vi "Pnuematic_Initialization.vi"   [LabVIEW 2018]
uses:
  <vilib>/Rock Robotics/WPI/Solenoid/WPI_SolenoidChannel.ctl
  <vilib>/Rock Robotics/WPI/Solenoid/WPI_SolenoidOpenDouble.vi
  <vilib>/Rock Robotics/WPI/Solenoid/WPI_SolenoidOpenSingle.vi
  Global_Variables/Refnum_Names.vi
  <vilib>/Rock Robotics/WPI/Utilities/WPI_GetSetVariantRefNum.vi
  Global_Variables/Elevator_Globals.vi
  Global_Variables/Intake_Disc_Globals.vi
  Global_Variables/Climb_Globals.vi
types:
  T1 = typedef "WPI_SolenoidChannel.ctl" = enum8{"Solenoid 0", "Solenoid 1", "Solenoid 2", "Solenoid 3", "Solenoid 4", "Solenoid 5", "Solenoid 6", "Solenoid 7", "Invalid"}
  T2 = typedef "WPI_SolenoidDevRef.ctl" = cluster{"DevStatus":errorcluster, "Pneumatics Control Module":u8, "Forward Solenoid Channel":T1, "Reverse Solenoid Channel":T1}
  T3 = typedef "WPI_CompressorDevRef.ctl" = cluster{"DevStatus":errorcluster, "Pneumatics Control Module":u8}
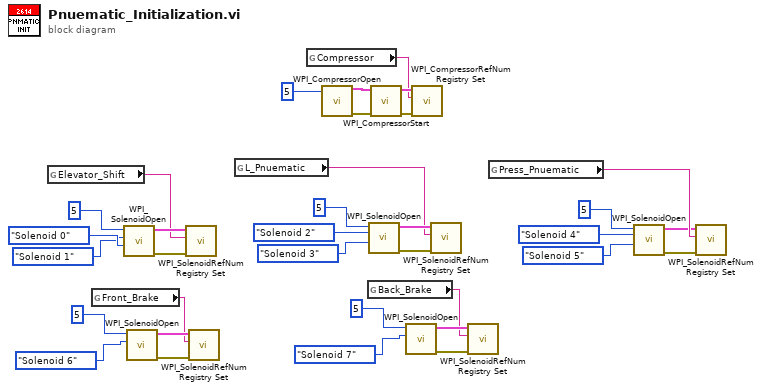
[diagram p0: block diagram]
diagram:
  n1 = global read "Elevator_Globals.vi" "Elevator_Shift"() -> (w10:string)
  n2 = global read "Elevator_Globals.vi" "Front_Brake"() -> (w8:string)
  n3 = call-poly <vilib>:"WPI_SolenoidOpen.vi"("Reverse Solenoid Channel"=WPI_SolenoidChannel."Solenoid 0", "Forward Solenoid Channel"=WPI_SolenoidChannel."Solenoid 1" ("Solenoid Channel"), "Pneumatics Control Module (0)"=u8 5) -> ("error out"=w24:errorcluster, "SolenoidDevRef"=w25:T2)  [unwired: 7 in]
  n4 = call-poly <vilib>:"WPI_SolenoidOpen.vi"("Solenoid Channel"=WPI_SolenoidChannel."Solenoid 6", "Pneumatics Control Module (0)"=u8 5) -> ("error out"=w15:errorcluster, "SolenoidDevRef"=w16:T2)  [unwired: 8 in]
  n5 = call <vilib>:"WPI_SolenoidRefNum Registry Set.vi"("error in (no error)"=w24, "refnum name"=w10, "SolenoidDevRef"=w25) -> ()  [unwired: 7 in, 2 out]
  n6 = call <vilib>:"WPI_SolenoidRefNum Registry Set.vi"("error in (no error)"=w15, "refnum name"=w8, "SolenoidDevRef"=w16) -> ()  [unwired: 7 in, 2 out]
  n7 = global read "Intake_Disc_Globals.vi" "L_Pnuematic"() -> (w9:string)
  n8 = global read "Refnum_Names.vi" "Compressor"() -> (w29:string)
  n9 = call <vilib>:"WPI_CompressorOpen.vi"("Pneumatics Control Module (0)"=u8 5) -> ("CompressorDevRef"=w33:T3, "error out"=w32:errorcluster)  [unwired: 13 in]
  n10 = global read "Climb_Globals.vi" "Back_Brake"() -> (w7:string)
  n11 = call-poly <vilib>:"WPI_SolenoidOpen.vi"("Reverse Solenoid Channel"=WPI_SolenoidChannel."Solenoid 3" ("Solenoid Channel"), "Forward Solenoid Channel"=WPI_SolenoidChannel."Solenoid 2" ("Reverse Solenoid Channel"), "Pneumatics Control Module (0)"=u8 5) -> ("error out"=w21:errorcluster, "SolenoidDevRef"=w22:T2)  [unwired: 7 in]
  n12 = call <vilib>:"WPI_CompressorStart.vi"("error in (no error)"=w32, "CompressorDevRef"=w33) -> ("error out"=w31:errorcluster, "CompressorDevRef"=w30:T3)  [unwired: 8 in]
  n13 = call-poly <vilib>:"WPI_SolenoidOpen.vi"("Solenoid Channel"=WPI_SolenoidChannel."Solenoid 7", "Pneumatics Control Module (0)"=u8 5) -> ("error out"=w14:errorcluster, "SolenoidDevRef"=w13:T2)  [unwired: 8 in]
  n14 = call <vilib>:"WPI_CompressorRefNum Registry Set.vi"("error in (no error)"=w31, "refnum name"=w29, "CompressorDevRef"=w30) -> ()  [unwired: 7 in, 2 out]
  n15 = call <vilib>:"WPI_SolenoidRefNum Registry Set.vi"("error in (no error)"=w21, "refnum name"=w9, "SolenoidDevRef"=w22) -> ()  [unwired: 7 in, 2 out]
  n16 = call <vilib>:"WPI_SolenoidRefNum Registry Set.vi"("error in (no error)"=w14, "refnum name"=w7, "SolenoidDevRef"=w13) -> ()  [unwired: 7 in, 2 out]
  n17 = global read "Intake_Disc_Globals.vi" "Press_Pnuematic"() -> (w6:string)
  n18 = call-poly <vilib>:"WPI_SolenoidOpen.vi"("Reverse Solenoid Channel"=WPI_SolenoidChannel."Solenoid 5" ("Solenoid Channel"), "Forward Solenoid Channel"=WPI_SolenoidChannel."Solenoid 4" ("Reverse Solenoid Channel"), "Pneumatics Control Module (0)"=u8 5) -> ("error out"=w3:errorcluster, "SolenoidDevRef"=w2:T2)  [unwired: 7 in]
  n19 = call <vilib>:"WPI_SolenoidRefNum Registry Set.vi"("error in (no error)"=w3, "refnum name"=w6, "SolenoidDevRef"=w2) -> ()  [unwired: 7 in, 2 out]
